vi "get data interface information.vi"(11 "Watchdog runtime in":refnum<class "Watchdog runtime.lvclass">) -> (2 "data type defs":T1, 3 "Watchdog runtime out":refnum<class "Watchdog runtime.lvclass">)   [LabVIEW 2013, in "Watchdog runtime.lvclass"]
uses:
  Watchdog runtime.lvclass
  <vilib>/NI/Tag Bus Data Framework/fixed module parent/module/execution/data cluster type definition.ctl
  output user data.ctl
  parameter user data.ctl
  result user data.ctl
  input user data.ctl
  <vilib>/NI/Tag Bus Data Framework/fixed module parent/module/execution/fixed channel runtime.lvclass
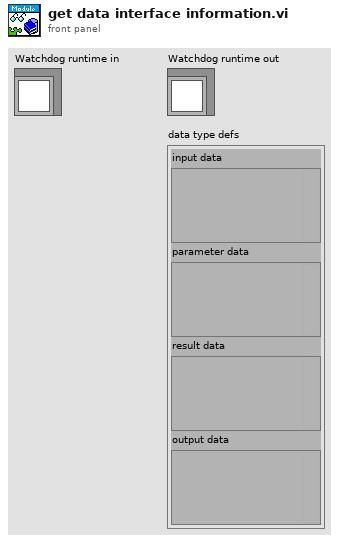
[diagram p1: front panel]
types:
  T1 = typedef "fixed channel runtime.lvclass/data cluster type definition.ctl" = cluster{"input data":variant, "parameter data":variant, "result data":variant, "output data":variant}
  T2 = typedef "Watchdog runtime.lvclass/input user data.ctl" = cluster{"placeholder":sgl}
  T3 = typedef "Watchdog runtime.lvclass/result user data.ctl" = cluster{"placeholder":sgl}
  T4 = typedef "Watchdog runtime.lvclass/parameter user data.ctl" = cluster{"placeholder":sgl}
  T5 = typedef "Watchdog runtime.lvclass/output user data.ctl" = cluster{"placeholder":sgl}
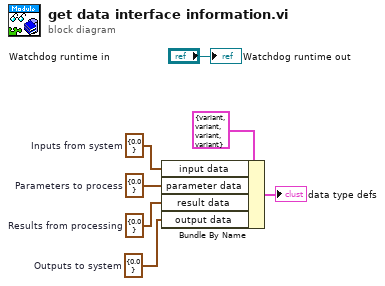
[diagram p0: block diagram]
diagram:
  w1 = T2 {"placeholder"=0.0}  # Inputs from system
  w3 = T3 {"placeholder"=0.0}  # Results from processing
  w2 = T4 {"placeholder"=0.0}  # Parameters to process
  w4 = T5 {"placeholder"=0.0}  # Outputs to system
  n1 = Bundle By Name(cluster=T1 {"input data"=variant, "parameter data"=variant, "result data"=variant, "output data"=variant} ("data type defs"), "input data"=w1, "parameter data"=w2, "result data"=w3, "output data"=w4) -> (→"data type defs":T1)
  "Watchdog runtime out" <- "Watchdog runtime in"
